vi "Read Single Measurement (Current Harmonics).vi"(0 "VISA resource name":refnum<visa-resource-name>, 5 "Maximum Time (10000 ms)":i32=10000, 7 "Harmonic Order (1)":u8=1, 9 "Phase Order (1)":u8=1, 11 "error in (no error)":errorcluster) -> (3 "Total Current Harmonic Distortion":dbl, 4 "VISA resource name out":refnum<visa-resource-name>, 6 "Current Crestfactor":dbl, 8 "Nth Current Harmonic Amplitude":dbl, 10 "Nth Current Harmonic Phase":dbl, 15 "error out":errorcluster)   [LabVIEW 2019, in "Agilent 681x Series.lvlib"]
doc: "Initiates the measurement and reads the selected order harmonic amplitude and phase values, the current crestfactor and the current total harmonic distortion.\n\n<B>Note:</B>\n\nThis VI changes the <B>Trigger Source</B> to <B>Bus</B> and uses a software trigger after the instrument is initiated. If you want to control the triggering and other features, please use the low level VIs."
uses:
  <instrlib>/Agilent 681x Series/Agilent 681x Series.lvlib
  <instrlib>/Agilent 681x Series/Public/Data/Low Level/Fetch Single Measurement (Current Harmonics).vi
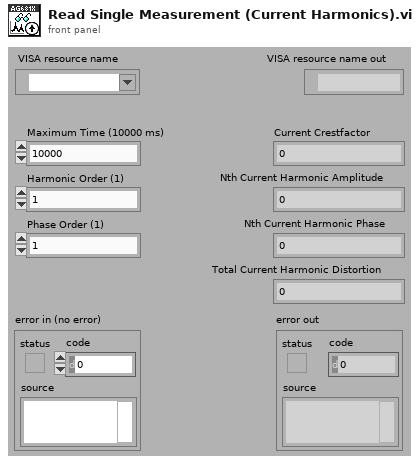
[diagram p1: front panel]
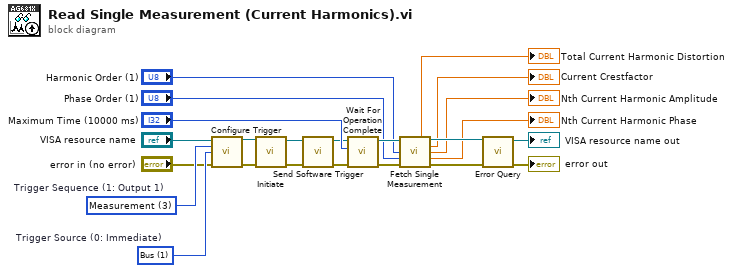
[diagram p0: block diagram]
diagram:
  w9 = 1 items=["Immediate", "Bus", "External", "Phase", "Trigger Out"]  # Trigger Source (0: Immediate)
  w10 = 3 items=["Output"=1, "Synchronous Source"=2, "Measurement"=3]  # Trigger Sequence (1: Output 1)
  n1 = call <instrlib>:"Configure Trigger.vi"("VISA resource name"="VISA resource name", "Trigger Sequence (1: Output 1)"=w10, "Trigger Source (0: Immediate)"=w9, "error in (no error)"="error in (no error)") -> ("VISA resource name out"=w7:refnum<visa-resource-name>, "error out"=w8:errorcluster)  [unwired: 10 in]
  n2 = call <instrlib>:"Initiate.vi"("error in (no error)"=w8, "VISA resource name"=w7) -> ("error out"=w6:errorcluster, "VISA resource name out"=w5:refnum<visa-resource-name>)  [unwired: 8 in]
  n3 = call <instrlib>:"Send Software Trigger.vi"("VISA resource name"=w5, "error in (no error)"=w6) -> ("VISA resource name out"=w3:refnum<visa-resource-name>, "error out"=w4:errorcluster)  [unwired: 12 in]
  n4 = call <instrlib>:"Wait For Operation Complete.vi"("error in (no error)"=w4, "Maximum Time (10000 ms)"="Maximum Time (10000 ms)", "VISA resource name"=w3) -> ("error out"=w22:errorcluster, "VISA resource name out"=w19:refnum<visa-resource-name>)  [unwired: 7 in]
  n5 = call-poly <instrlib>:"Fetch Single Measurement.vi"("VISA resource name"=w19, "Harmonic Order (1)"="Harmonic Order (1)", "Phase Order (1)"="Phase Order (1)", "error in (no error)"=w22) -> ("Total Current Harmonic Distortion"=→"Total Current Harmonic Distortion":dbl, "VISA resource name out"=w21:refnum<visa-resource-name>, "Current Crestfactor"=→"Current Crestfactor":dbl, "Nth Current Harmonic Amplitude"=→"Nth Current Harmonic Amplitude":dbl, "Nth Current Harmonic Phase"=→"Nth Current Harmonic Phase":dbl, "error out"=w20:errorcluster)  [unwired: 6 in]
  n6 = call <instrlib>:"Error Query.vi"("error in (no error)"=w20, "VISA resource name"=w21) -> ("error out"=→"error out":errorcluster, "VISA resource name out"=→"VISA resource name out":refnum<visa-resource-name>)  [unwired: 6 in, 2 out]
